vi "XYZ stage control.vi"() -> ()   [LabVIEW 2020]
panel:
  in  "Z down step size":dbl=100.0
  in  "Y down step size":dbl=100.0
  in  "X down step size":dbl=100.0
  out "X Position":dbl=-10.99177734375
  in  "X Step Size(um)":dbl=100.0
  in  "Right":bool
  in  "Left":bool
  out "Y Position":dbl=3.8870703125000023
  in  "Focus Down X":bool
  in  "Y Step Size(um)":dbl=100.0
  in  "Focus Up X":bool caption="Focus Up"
  in  "Focus Down":bool
  out "Z Position":dbl=6.860690000000502
  in  "Focus Up":bool
  in  "Z step size (um)":dbl=100.0
  in  "Close Communication":bool
  out "Error out":errorcluster
  out "Connected":bool=TRUE
  out "GetFirmwareVersion 2":string="3.03\r"
  in  "SPIIPLUSCOM660Lib.IAsyncChannel":refnum<k7>
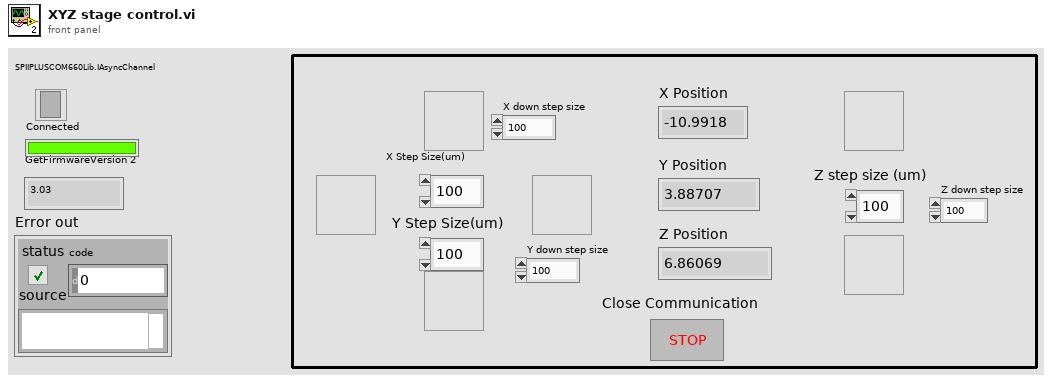
[diagram p1: front panel]
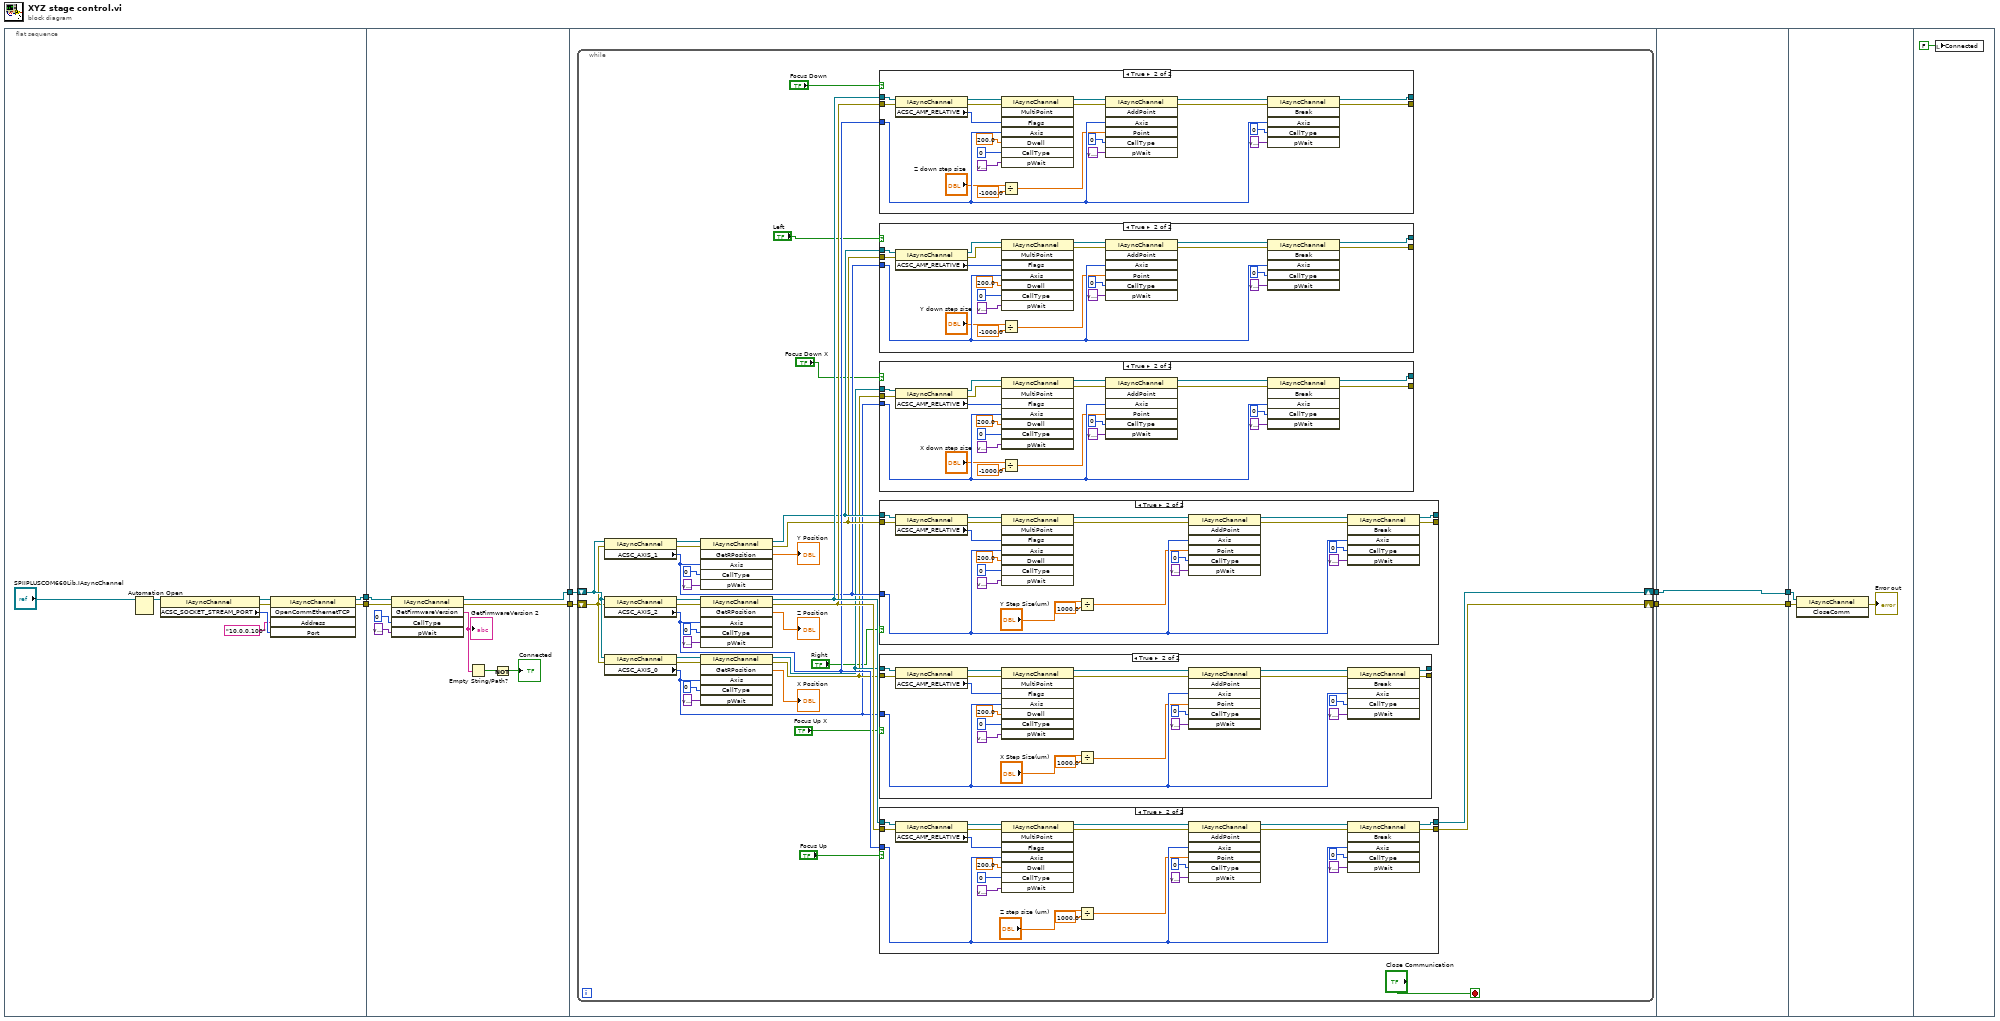
[diagram p0: block diagram]
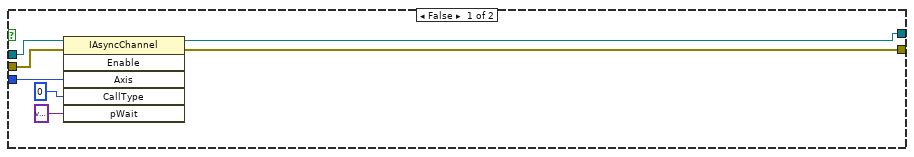
[diagram p2: hidden frame]
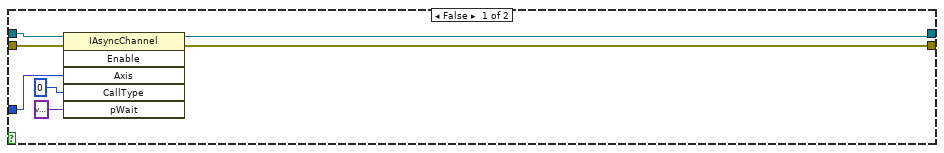
[diagram p3: hidden frame]
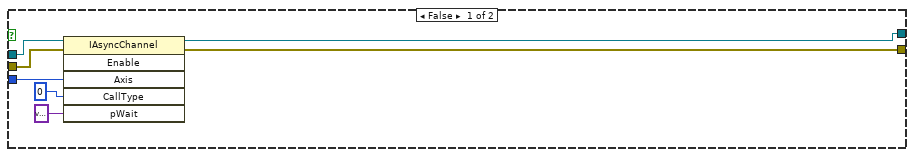
[diagram p4: hidden frame]
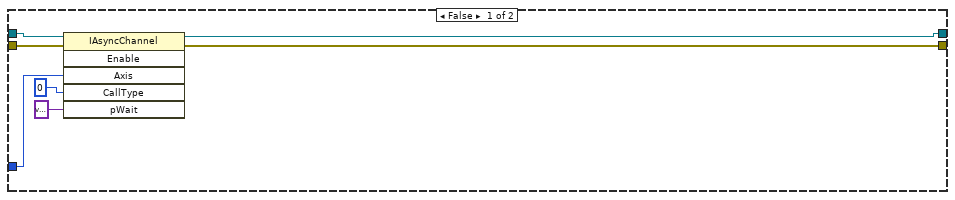
[diagram p5: hidden frame]
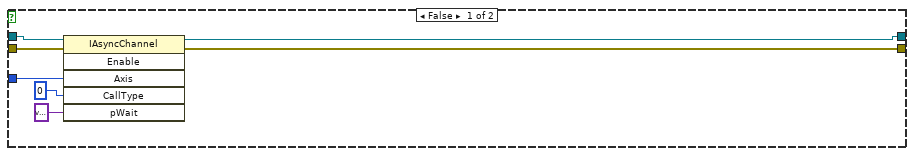
[diagram p6: hidden frame]
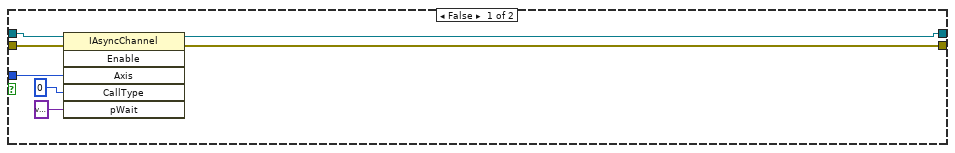
[diagram p7: hidden frame]
diagram:
  n1 = flat-sequence {
    tunnel: [w11] -> w8
    tunnel: [w10] -> w7
    tunnel: w8 -> [w21]
    tunnel: w7 -> [w20]
    tunnel: [w18] -> w6
    tunnel: [w17] -> w5
    tunnel: w6 -> [w26]
    tunnel: w5 -> [w29]
    tunnel: [w28] -> w4
    tunnel: [w27] -> w3
    tunnel: w4 -> [w240]
    tunnel: w3 -> [w239]
    tunnel: [w240] -> w2
    tunnel: [w239] -> w1
    tunnel: w2 -> [w242]
    tunnel: w1 -> [w241]
    frame #0 {
      n2 = Automation Open(Automation Refnum="SPIIPLUSCOM660Lib.IAsyncChannel") -> (Automation Refnum=w16:refnum<k7>)  [unwired: 3 in, 1 out]
      n3 = property class="IAsyncChannel"(reference=w16) -> (reference out=w15:refnum<k7>, error out=w9:errorcluster, "ACSC_SOCKET_STREAM_PORT"=w13:i32)  [unwired: 1 in]
      n4 = invoke class="IAsyncChannel" method="OpenCommEthernetTCP"(reference=w15, error in=w9, "Address"="10.0.0.100", "Port"=w13) -> (reference out=w11:refnum<k7>, error out=w10:errorcluster)  [unwired: 1 in, 3 out]
    }
    frame #1 {
      n5 = invoke class="IAsyncChannel" method="GetFirmwareVersion"(reference=w21, error in=w20, "CallType"=u64 0, "pWait"=variant) -> (reference out=w18:refnum<k7>, error out=w17:errorcluster, "GetFirmwareVersion"=w23:string)  [unwired: 1 in, 2 out]
      "GetFirmwareVersion 2" <- w23
      n6 = Empty String/Path?(string/path=w23) -> (empty?=w22:bool)
      n7 = Not(x=w22) -> (.not. x?=→"Connected":bool)
    }
    frame #2 {
      n8 = while {
        shift-right: [w64] -> w28
        shift-left: w26 -> [w43]
        shift-right: [w63] -> w27
        shift-left: w29 -> [w42]
        stop <- "Close Communication" stop-if-true
        n9 = property class="IAsyncChannel"(reference=w43, error in=w42) -> (reference out=w51:refnum<k7>, error out=w50:errorcluster, "ACSC_AXIS_1"=w47:i32)
        n10 = property class="IAsyncChannel"(reference=w43, error in=w42) -> (reference out=w60:refnum<k7>, error out=w59:errorcluster, "ACSC_AXIS_2"=w52:i32)
        n11 = property class="IAsyncChannel"(reference=w43, error in=w42) -> (reference out=w41:refnum<k7>, error out=w40:errorcluster, "ACSC_AXIS_0"=w36:i32)
        n12 = invoke class="IAsyncChannel" method="GetRPosition"(reference=w51, error in=w50, "Axis"=w47, "CallType"=u64 0, "pWait"=variant) -> (reference out=w49:refnum<k7>, error out=w48:errorcluster, "GetRPosition"=→"Y Position":dbl)  [unwired: 1 in, 3 out]
        n13 = invoke class="IAsyncChannel" method="GetRPosition"(reference=w60, error in=w59, "Axis"=w52, "CallType"=u64 0, "pWait"=variant) -> (reference out=w54:refnum<k7>, error out=w53:errorcluster, "GetRPosition"=→"Z Position":dbl)  [unwired: 1 in, 3 out]
        n14 = invoke class="IAsyncChannel" method="GetRPosition"(reference=w41, error in=w40, "Axis"=w36, "CallType"=u64 0, "pWait"=variant) -> (reference out=w38:refnum<k7>, error out=w37:errorcluster, "GetRPosition"=→"X Position":dbl)  [unwired: 1 in, 3 out]
        n15 = case shown="True" "Focus Down" {
          tunnel: w54 -> [w187 w208]
          tunnel: w53 -> [w186 w209]
          tunnel: [w185 w192] -> _
          tunnel: [w184 w191] -> _
          tunnel: w52 -> [w183 w195]
          frame False {
            n16 = invoke class="IAsyncChannel" method="Enable"(reference=w187, error in=w186, "Axis"=w183, "CallType"=u64 0, "pWait"=variant) -> (reference out=w185:refnum<k7>, error out=w184:errorcluster)  [unwired: 1 in, 4 out]
          }
          frame True {
            n17 = property class="IAsyncChannel"(reference=w208, error in=w209) -> (reference out=w207:refnum<k7>, error out=w206:errorcluster, "ACSC_AMF_RELATIVE"=w203:i32)
            n18 = invoke class="IAsyncChannel" method="MultiPoint"(reference=w207, error in=w206, "Flags"=w203, "Axis"=w195, "Dwell"=200.0, "CallType"=u64 0, "pWait"=variant) -> (reference out=w202:refnum<k7>, error out=w201:errorcluster)  [unwired: 1 in, 6 out]
            n19 = Divide(x="Z down step size", y=-1000.0) -> (x/y=w189:dbl)
            n20 = invoke class="IAsyncChannel" method="AddPoint"(reference=w202, error in=w201, "Axis"=w195, "Point"=w189, "CallType"=u64 0, "pWait"=variant) -> (reference out=w197:refnum<k7>, error out=w196:errorcluster)  [unwired: 1 in, 5 out]
            n21 = invoke class="IAsyncChannel" method="Break"(reference=w197, error in=w196, "Axis"=w195, "CallType"=u64 0, "pWait"=variant) -> (reference out=w192:refnum<k7>, error out=w191:errorcluster)  [unwired: 1 in, 4 out]
          }
        }
        n22 = case shown="True" "Left" {
          tunnel: w49 -> [w129 w150]
          tunnel: w48 -> [w128 w151]
          tunnel: [w127 w134] -> _
          tunnel: [w126 w133] -> _
          tunnel: w47 -> [w125 w137]
          frame False {
            n23 = invoke class="IAsyncChannel" method="Enable"(reference=w129, error in=w128, "Axis"=w125, "CallType"=u64 0, "pWait"=variant) -> (reference out=w127:refnum<k7>, error out=w126:errorcluster)  [unwired: 1 in, 4 out]
          }
          frame True {
            n24 = property class="IAsyncChannel"(reference=w150, error in=w151) -> (reference out=w149:refnum<k7>, error out=w148:errorcluster, "ACSC_AMF_RELATIVE"=w145:i32)
            n25 = invoke class="IAsyncChannel" method="MultiPoint"(reference=w149, error in=w148, "Flags"=w145, "Axis"=w137, "Dwell"=200.0, "CallType"=u64 0, "pWait"=variant) -> (reference out=w144:refnum<k7>, error out=w143:errorcluster)  [unwired: 1 in, 6 out]
            n26 = Divide(x="Y down step size", y=-1000.0) -> (x/y=w131:dbl)
            n27 = invoke class="IAsyncChannel" method="AddPoint"(reference=w144, error in=w143, "Axis"=w137, "Point"=w131, "CallType"=u64 0, "pWait"=variant) -> (reference out=w139:refnum<k7>, error out=w138:errorcluster)  [unwired: 1 in, 5 out]
            n28 = invoke class="IAsyncChannel" method="Break"(reference=w139, error in=w138, "Axis"=w137, "CallType"=u64 0, "pWait"=variant) -> (reference out=w134:refnum<k7>, error out=w133:errorcluster)  [unwired: 1 in, 4 out]
          }
        }
        n29 = case shown="True" "Focus Down X" {
          tunnel: w38 -> [w71 w92]
          tunnel: w37 -> [w70 w93]
          tunnel: [w69 w76] -> _
          tunnel: [w68 w75] -> _
          tunnel: w36 -> [w67 w79]
          frame False {
            n30 = invoke class="IAsyncChannel" method="Enable"(reference=w71, error in=w70, "Axis"=w67, "CallType"=u64 0, "pWait"=variant) -> (reference out=w69:refnum<k7>, error out=w68:errorcluster)  [unwired: 1 in, 4 out]
          }
          frame True {
            n31 = property class="IAsyncChannel"(reference=w92, error in=w93) -> (reference out=w91:refnum<k7>, error out=w90:errorcluster, "ACSC_AMF_RELATIVE"=w87:i32)
            n32 = invoke class="IAsyncChannel" method="MultiPoint"(reference=w91, error in=w90, "Flags"=w87, "Axis"=w79, "Dwell"=200.0, "CallType"=u64 0, "pWait"=variant) -> (reference out=w86:refnum<k7>, error out=w85:errorcluster)  [unwired: 1 in, 6 out]
            n33 = Divide(x="X down step size", y=-1000.0) -> (x/y=w73:dbl)
            n34 = invoke class="IAsyncChannel" method="AddPoint"(reference=w86, error in=w85, "Axis"=w79, "Point"=w73, "CallType"=u64 0, "pWait"=variant) -> (reference out=w81:refnum<k7>, error out=w80:errorcluster)  [unwired: 1 in, 5 out]
            n35 = invoke class="IAsyncChannel" method="Break"(reference=w81, error in=w80, "Axis"=w79, "CallType"=u64 0, "pWait"=variant) -> (reference out=w76:refnum<k7>, error out=w75:errorcluster)  [unwired: 1 in, 4 out]
          }
        }
        n36 = case shown="True" "Right" {
          tunnel: w49 -> [w158 w179]
          tunnel: w48 -> [w157 w180]
          tunnel: [w156 w163] -> _
          tunnel: [w155 w162] -> _
          tunnel: w47 -> [w154 w166]
          frame False {
            n37 = invoke class="IAsyncChannel" method="Enable"(reference=w158, error in=w157, "Axis"=w154, "CallType"=u64 0, "pWait"=variant) -> (reference out=w156:refnum<k7>, error out=w155:errorcluster)  [unwired: 1 in, 4 out]
          }
          frame True {
            n38 = property class="IAsyncChannel"(reference=w179, error in=w180) -> (reference out=w178:refnum<k7>, error out=w177:errorcluster, "ACSC_AMF_RELATIVE"=w174:i32)
            n39 = invoke class="IAsyncChannel" method="MultiPoint"(reference=w178, error in=w177, "Flags"=w174, "Axis"=w166, "Dwell"=200.0, "CallType"=u64 0, "pWait"=variant) -> (reference out=w173:refnum<k7>, error out=w172:errorcluster)  [unwired: 1 in, 6 out]
            n40 = Divide(x="Y Step Size(um)", y=1000.0) -> (x/y=w160:dbl)
            n41 = invoke class="IAsyncChannel" method="AddPoint"(reference=w173, error in=w172, "Axis"=w166, "Point"=w160, "CallType"=u64 0, "pWait"=variant) -> (reference out=w168:refnum<k7>, error out=w167:errorcluster)  [unwired: 1 in, 5 out]
            n42 = invoke class="IAsyncChannel" method="Break"(reference=w168, error in=w167, "Axis"=w166, "CallType"=u64 0, "pWait"=variant) -> (reference out=w163:refnum<k7>, error out=w162:errorcluster)  [unwired: 1 in, 4 out]
          }
        }
        n43 = case shown="True" "Focus Up X" {
          tunnel: w38 -> [w100 w121]
          tunnel: w37 -> [w99 w122]
          tunnel: [w98 w105] -> _
          tunnel: [w97 w104] -> _
          tunnel: w36 -> [w96 w108]
          frame False {
            n44 = invoke class="IAsyncChannel" method="Enable"(reference=w100, error in=w99, "Axis"=w96, "CallType"=u64 0, "pWait"=variant) -> (reference out=w98:refnum<k7>, error out=w97:errorcluster)  [unwired: 1 in, 4 out]
          }
          frame True {
            n45 = property class="IAsyncChannel"(reference=w121, error in=w122) -> (reference out=w120:refnum<k7>, error out=w119:errorcluster, "ACSC_AMF_RELATIVE"=w116:i32)
            n46 = invoke class="IAsyncChannel" method="MultiPoint"(reference=w120, error in=w119, "Flags"=w116, "Axis"=w108, "Dwell"=200.0, "CallType"=u64 0, "pWait"=variant) -> (reference out=w115:refnum<k7>, error out=w114:errorcluster)  [unwired: 1 in, 6 out]
            n47 = Divide(x="X Step Size(um)", y=1000.0) -> (x/y=w102:dbl)
            n48 = invoke class="IAsyncChannel" method="AddPoint"(reference=w115, error in=w114, "Axis"=w108, "Point"=w102, "CallType"=u64 0, "pWait"=variant) -> (reference out=w110:refnum<k7>, error out=w109:errorcluster)  [unwired: 1 in, 5 out]
            n49 = invoke class="IAsyncChannel" method="Break"(reference=w110, error in=w109, "Axis"=w108, "CallType"=u64 0, "pWait"=variant) -> (reference out=w105:refnum<k7>, error out=w104:errorcluster)  [unwired: 1 in, 4 out]
          }
        }
        n50 = case shown="True" "Focus Up" {
          tunnel: w54 -> [w216 w237]
          tunnel: w53 -> [w215 w238]
          tunnel: [w214 w221] -> w64
          tunnel: [w213 w220] -> w63
          tunnel: w52 -> [w212 w224]
          frame False {
            n51 = invoke class="IAsyncChannel" method="Enable"(reference=w216, error in=w215, "Axis"=w212, "CallType"=u64 0, "pWait"=variant) -> (reference out=w214:refnum<k7>, error out=w213:errorcluster)  [unwired: 1 in, 4 out]
          }
          frame True {
            n52 = property class="IAsyncChannel"(reference=w237, error in=w238) -> (reference out=w236:refnum<k7>, error out=w235:errorcluster, "ACSC_AMF_RELATIVE"=w232:i32)
            n53 = invoke class="IAsyncChannel" method="MultiPoint"(reference=w236, error in=w235, "Flags"=w232, "Axis"=w224, "Dwell"=200.0, "CallType"=u64 0, "pWait"=variant) -> (reference out=w231:refnum<k7>, error out=w230:errorcluster)  [unwired: 1 in, 6 out]
            n54 = Divide(x="Z step size (um)", y=1000.0) -> (x/y=w218:dbl)
            n55 = invoke class="IAsyncChannel" method="AddPoint"(reference=w231, error in=w230, "Axis"=w224, "Point"=w218, "CallType"=u64 0, "pWait"=variant) -> (reference out=w226:refnum<k7>, error out=w225:errorcluster)  [unwired: 1 in, 5 out]
            n56 = invoke class="IAsyncChannel" method="Break"(reference=w226, error in=w225, "Axis"=w224, "CallType"=u64 0, "pWait"=variant) -> (reference out=w221:refnum<k7>, error out=w220:errorcluster)  [unwired: 1 in, 4 out]
          }
        }
      }
    }
    frame #3 {
    }
    frame #4 {
      n57 = invoke class="IAsyncChannel" method="CloseComm"(reference=w242, error in=w241) -> (error out=→"Error out":errorcluster)  [unwired: 1 in, 2 out]
    }
    frame #5 {
      n58 = local write "Connected"(FALSE ("Connected")) -> ()
    }
  }
